vi "KML-Log.vi"(4 "path to vi or exe (in)":path, 5 "Tilt":string="0", 6 "Heading":string="0", 7 "Range":string="1500", 8 "Coords (in)":string, 9 "TimerIN (sh)":u32, 10 "WriteToFile?":bool, 11 "data in":string) -> (1 "Cur loc (out)":string, 3 "Timer OUT (sh)":u32)   [LabVIEW 8.6]
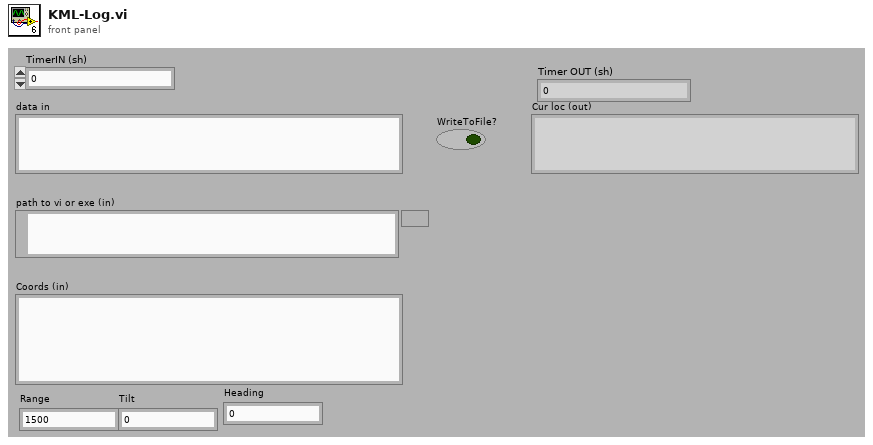
[diagram p1: front panel]
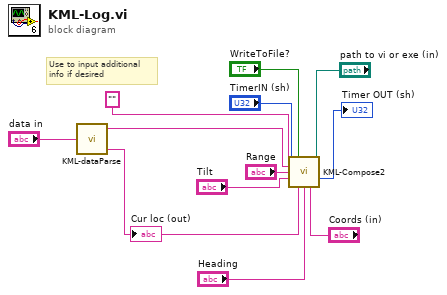
[diagram p0: block diagram]
diagram:
  # "Use to input additional\ninfo if desired"
  n1 = call "KML-dataParse.vi"("data in"="data in") -> ("ALT"=w9:string, "Cur loc (out)"=w4:string)  [unwired: 1 in]
  "Cur loc (out)" <- w4
  n2 = call "KML-Compose2.vi"("TimerIN (sh)"="TimerIN (sh)", "WriteToFile?"="WriteToFile?", "SPD"="", "path to vi or exe"="path to vi or exe (in)", "ALT"=w9, "Range"="Range", "Tilt"="Tilt", "Current Location"=w4, "Heading"="Heading", "Coords"="Coords (in)") -> ("Timer OUT (sh)"=→"Timer OUT (sh)":u32)  [unwired: 4 in, 1 out]
